vi "Indicator Init.vi"(7 "VolatusAPI":refnum<class "VolatusAPI.lvclass">, 8 "error in (no error)":errorcluster, 10 "JSON":string, 11 "NumericIndicator in":refnum<class "NumericIndicator.lvclass">) -> (0 "error out":errorcluster, 3 "NumericIndicator out":refnum<class "NumericIndicator.lvclass">)   [LabVIEW 2020, in "VolatusGUI.lvlib" / "NumericIndicator.lvclass"]
uses:
  NumericIndicator.lvclass
  NumericIndicator.lvclass/NumericIndicator.ctl
  JSON.ctl
  bc1d0ba6-3274-416f-84ea-d61b916d66ff.vi
  lv-vecto/Vecto/Group/Group.lvclass
  Volatus/VolatusAPI/VolatusAPI.lvclass
  C:/dev/lv20CE/relink/lv-vecto/Vecto/GroupAbstract/GroupAbstract.lvclass
  C:/dev/lv20CE/relink/lv-vecto/Vecto/Group/Group.lvclass
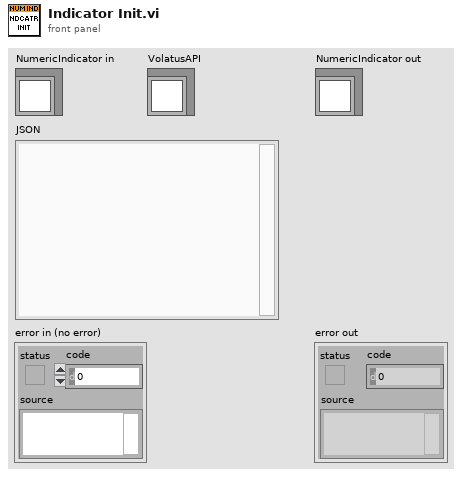
[diagram p1: front panel]
types:
  T1 = typedef "VolatusGUI.lvlib/NumericIndicator.lvclass/JSON.ctl" = cluster{"Group":string, "Channel":string}
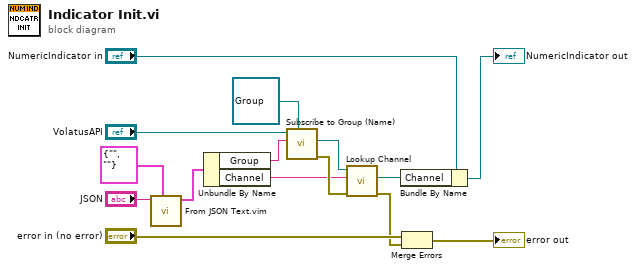
[diagram p0: block diagram]
diagram:
  n1 = call "From JSON Text.vim"("Data Type and Default Value"=T1 {"Group"="", "Channel"=""} ("JSON"), "JSON"="JSON") -> ("Data out"=w10:T1)  [unwired: 8 in, 1 out]
  n2 = Unbundle By Name(w10) -> ("Group"=w3:string, "Channel"=w9:string)
  n3 = call "Subscribe to Group (Name).vi"("Group Type"=refnum<class "Group.lvclass"> refnum ("Group in"), "Group Name"=w3, "VolatusAPI in"="VolatusAPI") -> ("error out"=w15:errorcluster, "Group"=w1:refnum<class "Group.lvclass">)  [unwired: 6 in, 1 out]
  n4 = call "Lookup Channel.vi"("error in (no error)"=w15, "Channel Name"=w9, "Group in"=w1) -> ("error out"=w5:errorcluster, "Channel"=w7:refnum<class "Channel.lvclass">)  [unwired: 6 in, 1 out]
  n5 = Bundle By Name(cluster="NumericIndicator in", "Channel"=w7) -> (→"NumericIndicator out":refnum<class "NumericIndicator.lvclass">)
  n6 = Merge Errors("error in (no error)", w5) -> (→"error out":errorcluster)
